vi "Waveform SimulatorOriginal.vi"(9 "Waveform Parameters":T2={"Frequency"=50.0, "Amplitude"=5.0, "Shape"=enum."Sine"}, 10 "Digitizing Parameters":T1={"Numbers of Samples"=100, "Sampling Frequency"=1000.0}) -> (2 "Waveform Output":cluster{"Time":dbl[], "Displacement":dbl[]} {"Time" format="%.10g"; "Displacement" format="%.6g"})   [LabVIEW 2017]
uses:
  <vilib>/imath/engines/lvmath2/RunTimeEngine/Managers/WorkSpace/UID Generator.vi
  <vilib>/imath/engines/lvmath2/RunTimeEngine/RunTimeType/NIMS_RunTimeType_From StrictType (excl LVString).vi
  <instcachedir>/0/NIMS_RunTimeType_From StrictType (excl LVString)_1019F277F0A747EDBCA0F6C52CA54500.lvgen/NIMS_RunTimeType_From StrictType (excl LVString)_1019F277F0A747EDBCA0F6C52CA54500_000.vi
  <vilib>/imath/engines/lvmath2/RunTimeEngine/LocalVariableDefStatement/MC_LocalVariableDefStatement_Display.vi
  <vilib>/imath/engines/lvmath2/RunTimeEngine/RangeToken/NIMS_Range.vi
  <instcachedir>/0/NIMS_Range_69CB9AAD882742A19CF7E739BE79952C.lvgen/NIMS_Range_69CB9AAD882742A19CF7E739BE79952C_000.vi
  <vilib>/imathl/engines/lvmath/Functions/Error Handling/Create Error.vi
  <vilib>/imath/engines/lvmath2/RunTimeEngine/ArithmeticOperatorToken/NIMS_ArithmeticOperator_plus.vi
  <instcachedir>/0/NIMS_ArithmeticOperator_plus_9255C7DA94A9479C92F91DC2DA9A664F.lvgen/NIMS_ArithmeticOperator_plus_9255C7DA94A9479C92F91DC2DA9A664F_004.vi
  <vilib>/imath/engines/lvmath2/RunTimeEngine/BuiltInFunctions/gensignal/NIMS_gensignal(str,RS,RS,RS).vi
  <vilib>/imath/engines/lvmath2/RunTimeEngine/BuiltInFunctions/transpose/NIMS_transpose(GV).vi
  <instcachedir>/0/NIMS_transpose(GV)_1D76875BF542458FA31D2D0CC3E998C0.lvgen/NIMS_transpose(GV)_1D76875BF542458FA31D2D0CC3E998C0_000.vi
  <vilib>/imath/engines/lvmath2/RunTimeEngine/BuiltInFunctions/linramp/NIMS_linramp.vi
  <vilib>/imath/engines/lvmath2/RunTimeEngine/VariableToken/NIMS_VariableToken_CondDefined.vi
  <instcachedir>/0/NIMS_VariableToken_CondDefined_6E7F1EE7F80E48298C84CF05BD736261.lvgen/NIMS_VariableToken_CondDefined_6E7F1EE7F80E48298C84CF05BD736261_003.vi
  <vilib>/imath/engines/lvmath/Functions/Error Handling/MergeErrorsWrapper.vi
  <vilib>/imath/engines/lvmath2/RunTimeEngine/Managers/SymbolTable/Clear UID.vi
  <vilib>/imath/engines/lvmath2/RunTimeEngine/NodeEndStatement/NIMS_NodeEndStatement_Output.vi
  <instcachedir>/0/NIMS_NodeEndStatement_Output_53EC0D466D134D7ABD903AC30B43404B.lvgen/NIMS_NodeEndStatement_Output_53EC0D466D134D7ABD903AC30B43404B_005.vi
  <vilib>/imath/engines/lvmath2/RunTimeEngine/ErrorHandling/NIMS_Finalize Error.vi
  <vilib>/imath/engines/lvmath2/RunTimeEngine/Managers/SymbolTable/NIMS_WorkSpace.lvlib
panel:
  in  "Tab Control":enum32{"Page 1", "Page 2", "Page 3"}(tab)
  out "XY Graph":cluster{"t":dbl[], "x":dbl[]}(graph)
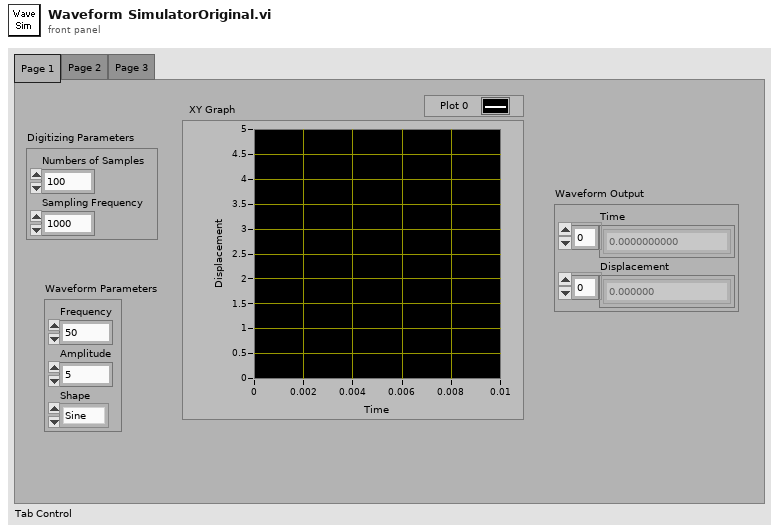
[diagram p1: front panel]
types:
  T1 = cluster{"Numbers of Samples":i32, "Sampling Frequency":dbl}
  T2 = cluster{"Frequency":dbl, "Amplitude":dbl, "Shape":enum16{"Sine", "Cosine", "DC Level", "Square", "User-Defined"}}
  T3 = enum16{"Sine", "Cosine", "DC Level", "Square", "User-Defined"}
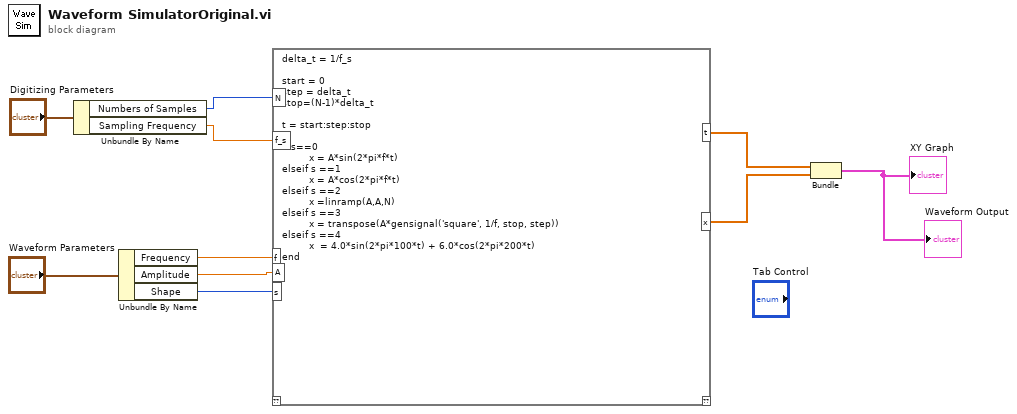
[diagram p0: block diagram]
diagram:
  n1 = Unbundle By Name("Digitizing Parameters") -> ("Numbers of Samples"=w4:i32, "Sampling Frequency"=w5:dbl)
  n2 = Unbundle By Name("Waveform Parameters") -> ("Frequency"=w8:dbl, "Amplitude"=w9:dbl, "Shape"=w10:T3)
  n3 = mathscript code="delta_t = 1/f_s\n\nstart = 0\nstep = delta_t\nstop=(N-1)*delta_t\n\nt = start:step:stop\n\nif s==0\n         x = A*sin(2*pi*f*t)\nelseif s ==1\n         x = A*cos(2*pi*f*t)\nelseif s ==2\n         x =linramp(A,A,N)\nelseif s ==3\n         x = transpose(A*gensignal('square', 1/f, stop, step))\nelseif s ==4\n         x  = 4.0*sin(2*pi*100*t) + 6.0*cos(2*pi*200*t)\nend"("N"=w4, "f_s"=w5, "f"=w8, "A"=w9, "s"=w10) -> ("t"=w1:dbl[], "x"=w2:dbl[])  [unwired: 1 in, 1 out]
  n4 = Bundle("t"=w1, "x"=w2) -> (→"XY Graph" →"Waveform Output":cluster{"t":dbl[], "x":dbl[]})  [unwired: 1 in]
